vi "ITX to TDMS.vi"(8 "error in (no error)":errorcluster, 10 "file (use dialog)":path=path "P:/sample/GaAs/GaAs quantum dots/2008/PL Map/A1 735/060731ASBA_A1_6.0.itx", 11 "LVtoITX in":refnum<class "LV to ITX.lvclass">) -> (0 "error out":errorcluster, 3 "LVtoITX out":refnum<class "LV to ITX.lvclass">)   [LabVIEW 2016, in "LV to ITX.lvclass"]
uses:
  LV to ITX.lvclass
  LV to ITX.lvclass/LV to ITX.ctl
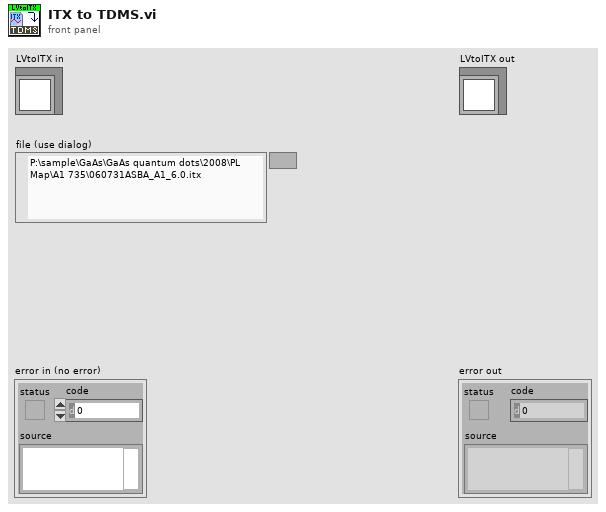
[diagram p1: front panel]
types:
  T1 = typedef "LV to ITX.lvclass/Dictionary--cluster.ctl" = cluster{"key":string, "value":variant}
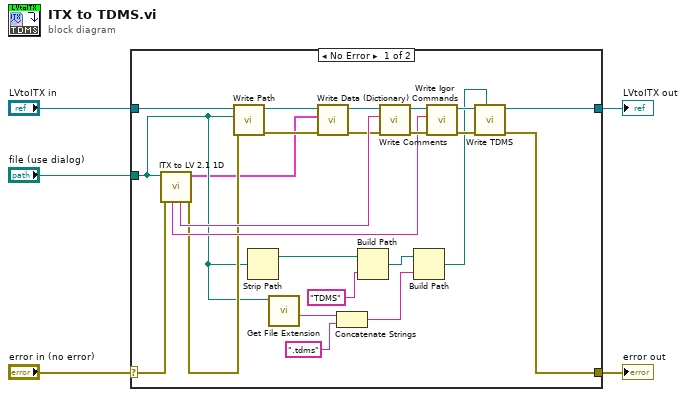
[diagram p0: block diagram]
diagram:
  n1 = case shown="No Error" "error in (no error)" {
    selector: "error in (no error)" -> [w29 w31]
    tunnel: [w18 w31] -> w4
    tunnel: [w17 w30] -> w2
    tunnel: "LVtoITX in" -> [w27 w30]
    tunnel: "file (use dialog)" -> [w14 _]
    frame No Error {
      n2 = call "ITX to LV 2.1 1D.vi"("error in"=w29, "file (use dialog)"=w14) -> ("error out"=w19:errorcluster, "Data (Dictionary)"=w7:T1[], "Notes"=w28:string, "Commands"=w22:string)  [unwired: 4 in, 2 out]
      n3 = call "Write Path.vi"("error in (no error)"=w19, "Path"=w14, "LVtoITX in"=w27) -> ("error out"=w25:errorcluster, "LVtoITX out"=w26:refnum<class "LV to ITX.lvclass">)  [unwired: 7 in]
      n4 = Strip Path(path=w14) -> (stripped path=w10:path)  [unwired: 1 out]
      n5 = call <vilib>:"Get File Extension.vi"("file"=w14) -> ("filename without extension"=w16:string)  [unwired: 6 in, 4 out]
      n6 = call "Write Data (Dictionary).vi"("error in (no error)"=w25, "Data (Dictionary)"=w7, "LVtoITX in"=w26) -> ("error out"=w8:errorcluster, "LVtoITX out"=w9:refnum<class "LV to ITX.lvclass">)  [unwired: 7 in]
      n7 = Concatenate Strings(w16, ".tdms" ("string")) -> (w15:string)
      n8 = Build Path(base path=w10, name or relative path="TDMS" ("string")) -> (appended path=w11:path)
      n9 = call "Write Comments.vi"("error in (no error)"=w8, "Comments"=w28, "LVtoITX in"=w9) -> ("error out"=w23:errorcluster, "LVtoITX out"=w24:refnum<class "LV to ITX.lvclass">)  [unwired: 7 in]
      n10 = Build Path(base path=w11, name or relative path=w15) -> (appended path=w6:path)
      n11 = call "Write Igor Commands.vi"("error in (no error)"=w23, "Igor Commands"=w22, "LVtoITX in"=w24) -> ("error out"=w20:errorcluster, "LVtoITX out"=w21:refnum<class "LV to ITX.lvclass">)  [unwired: 7 in]
      n12 = call "Write TDMS.vi"("path"=w6, "error in (no error)"=w20, "LVtoITX in"=w21) -> ("error out"=w18:errorcluster, "LVtoITX out"=w17:refnum<class "LV to ITX.lvclass">)  [unwired: 6 in, 1 out]
    }
    frame Error {
    }
  }
  "error out" <- w4
  "LVtoITX out" <- w2
